vi "Simple Data Client.vi"() -> ()   [LabVIEW 2015]
doc: "This VI displays information transmitted by the Simple Data Server.vi. Set the Address control to the IP address of the RT target device. Set the Port control to the same value as the Port on the server. Be sure to start Simple Data Server before starting this client VI."
panel:
  in  "stop":bool
  out "chart":dbl[](graph)
  in  "Target IP Address":string="172.22.11.2"
  in  "Port":u16=2055 min=1025 step=1
  # "This VI displays information transmitted by the Simple Data Server.vi.  \nSet the Target IP Address control to the IP address of your evaluation \nkit. Set the Port control to the same value as the Port on the server.  \nStart Simple Data Server.vi before starting this client VI."
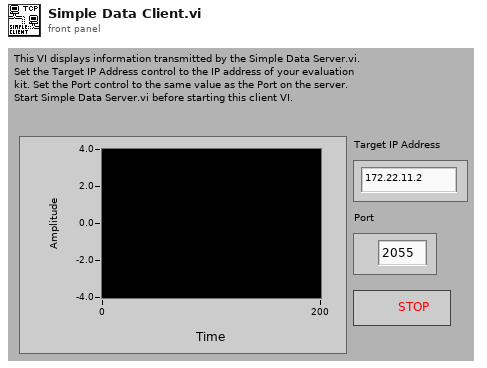
[diagram p1: front panel]
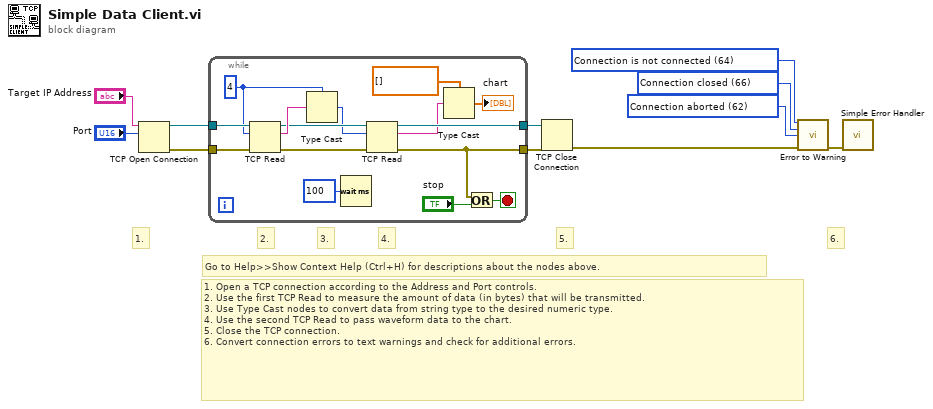
[diagram p0: block diagram]
diagram:
  w1 = 62 items=["No Error", "Argument Error", "Memory Full", "Out of Zone", "End of File", "File Already Open", "Generic File IO Error", "File Not Found", "File Permission Error", "Disk Full", "Duplicate Path", "Too Many Files Open", "Not Enabled", "Resource File Not Found", "Cannot Add Resource", "Resource Not Found", "Image Not Found", "Image Memory Error", "Pen Does Not Exist", "Config Bad Type", "Config Token Not Found", "Config Parse Error", "Config Memory Error", "Bad External Code Format", "Bad External Code Offset", "External Code Not Present", "Null Window", "Destroy Window Mixup", "Null Menu", "Print Aborted", "Bad Print Record", "Print Driver Error", "Windows Error During Print", "Memory Error During Print", "Print Dialog Error", "Generic Print Error", "Invalid Device Refnum", "Device Not Found", "Device Parameter Error", "Device Unit Error", "Can't Open Device", "Device Call Aborted", "Generic Error", "Cancelled By User", "Object ID Too Low", "Object ID Too High", "Object Not In Heap", "Unknown Heap", "Bad DefProc ID", "DefProc Not In Table", "Message Out Of Range", "Null Method", "Unknown Message", "Manager Call Not Supported", "Bad address", "Connection In progress", "Connection timed out", "Connection is already in progress", "Network attribute not supported", "Network error", "Address in use", "System out of memory", "Connection aborted", "Connection refused", "Connection is not connected", "Connection is already connected", "Connection closed", "Initialize error (interapplication manager)", "Bad occurrence", "Wait on unbound occurrence handler", "Occurrence queue overflow", "Bad path", "Semaphore not signaled", "Unrecognized type (interapplication manager)"] ("1st Error to Convert")
  w2 = 66 items=["No Error", "Argument Error", "Memory Full", "Out of Zone", "End of File", "File Already Open", "Generic File IO Error", "File Not Found", "File Permission Error", "Disk Full", "Duplicate Path", "Too Many Files Open", "Not Enabled", "Resource File Not Found", "Cannot Add Resource", "Resource Not Found", "Image Not Found", "Image Memory Error", "Pen Does Not Exist", "Config Bad Type", "Config Token Not Found", "Config Parse Error", "Config Memory Error", "Bad External Code Format", "Bad External Code Offset", "External Code Not Present", "Null Window", "Destroy Window Mixup", "Null Menu", "Print Aborted", "Bad Print Record", "Print Driver Error", "Windows Error During Print", "Memory Error During Print", "Print Dialog Error", "Generic Print Error", "Invalid Device Refnum", "Device Not Found", "Device Parameter Error", "Device Unit Error", "Can't Open Device", "Device Call Aborted", "Generic Error", "Cancelled By User", "Object ID Too Low", "Object ID Too High", "Object Not In Heap", "Unknown Heap", "Bad DefProc ID", "DefProc Not In Table", "Message Out Of Range", "Null Method", "Unknown Message", "Manager Call Not Supported", "Bad address", "Connection In progress", "Connection timed out", "Connection is already in progress", "Network attribute not supported", "Network error", "Address in use", "System out of memory", "Connection aborted", "Connection refused", "Connection is not connected", "Connection is already connected", "Connection closed", "Initialize error (interapplication manager)", "Bad occurrence", "Wait on unbound occurrence handler", "Occurrence queue overflow", "Bad path", "Semaphore not signaled", "Unrecognized type (interapplication manager)"] ("1st Error to Convert")
  w3 = 64 items=["No Error", "Argument Error", "Memory Full", "Out of Zone", "End of File", "File Already Open", "Generic File IO Error", "File Not Found", "File Permission Error", "Disk Full", "Duplicate Path", "Too Many Files Open", "Not Enabled", "Resource File Not Found", "Cannot Add Resource", "Resource Not Found", "Image Not Found", "Image Memory Error", "Pen Does Not Exist", "Config Bad Type", "Config Token Not Found", "Config Parse Error", "Config Memory Error", "Bad External Code Format", "Bad External Code Offset", "External Code Not Present", "Null Window", "Destroy Window Mixup", "Null Menu", "Print Aborted", "Bad Print Record", "Print Driver Error", "Windows Error During Print", "Memory Error During Print", "Print Dialog Error", "Generic Print Error", "Invalid Device Refnum", "Device Not Found", "Device Parameter Error", "Device Unit Error", "Can't Open Device", "Device Call Aborted", "Generic Error", "Cancelled By User", "Object ID Too Low", "Object ID Too High", "Object Not In Heap", "Unknown Heap", "Bad DefProc ID", "DefProc Not In Table", "Message Out Of Range", "Null Method", "Unknown Message", "Manager Call Not Supported", "Bad address", "Connection In progress", "Connection timed out", "Connection is already in progress", "Network attribute not supported", "Network error", "Address in use", "System out of memory", "Connection aborted", "Connection refused", "Connection is not connected", "Connection is already connected", "Connection closed", "Initialize error (interapplication manager)", "Bad occurrence", "Wait on unbound occurrence handler", "Occurrence queue overflow", "Bad path", "Semaphore not signaled", "Unrecognized type (interapplication manager)"] ("1st Error to Convert")
  # "Go to Help>>Show Context Help (Ctrl+H) for descriptions about the nodes above."
  # "6."
  # "5."
  # "4."
  # "3."
  # "2."
  # "1."
  # "1. Open a TCP connection according to the Address and Port controls.\n2. Use the first TCP Read to measure the amount of data (in bytes) that will be transmitted.\n3. Use Type Cast nodes to convert data from string type to the desired numeric type.\n4. Use the second TCP Read to pass waveform data to the chart.\n5. Close the TCP connection.\n6. Convert connection errors to text warnings and check for additional errors."
  n1 = TCP Open Connection(address="Target IP Address", remote port or service name="Port") -> (connection ID=w7:refnum<k5>, error out=w6:errorcluster)  [unwired: 1 in, 2 out]
  n2 = while {
    tunnel: w6 -> [w20]
    tunnel: w7 -> [w21]
    tunnel: [w22] -> w8
    tunnel: [w12] -> w9
    stop <- w16 stop-if-true
    w18 = 4
    n3 = TCP Read(connection ID=w21, bytes to read=w18, error in (no error)=w20) -> (connection ID out=w25:refnum<k5>, data out=w26:string, error out=w24:errorcluster)  [unwired: 2 out]
    n4 = Type Cast(type=w18, x=w26) -> (*(type *) &x=w23:i32)
    n5 = Wait (ms)(milliseconds to wait=u32 100) -> ()  [unwired: 1 out]
    n6 = TCP Read(connection ID=w25, bytes to read=w23, error in (no error)=w24) -> (connection ID out=w22:refnum<k5>, data out=w19:string, error out=w12:errorcluster)  [unwired: 2 out]
    n7 = Type Cast(type=dbl[] [] ("chart"), x=w19) -> (*(type *) &x=→"chart":dbl[])
    n8 = Or(x=w12, y="stop") -> (x .or. y?=w16:bool)
  }
  n9 = TCP Close Connection(connection ID=w8, error in (no error)=w9) -> (error out=w5:errorcluster)  [unwired: 2 out]
  n10 = call <vilib>:"Error to Warning.vi"("1st Error to Convert"=w3, "2nd Error to Convert"=w2, "3rd Error to Convert"=w1, "error in"=w5) -> ("warning out"=w4:errorcluster)  [unwired: 2 in, 9 out]
  n11 = call <vilib>:"Simple Error Handler.vi"("error in (no error)"=w4) -> ()  [unwired: 1 in, 8 out]
